vi "fpga_status.vi"(8 "error in (no error)":errorcluster, 11 "5785_2_x_200MHz in":refnum<class "5785_2_x_200MHz.lvclass">) -> (0 "error out":errorcluster, 2 "pulse TX status":T1, 3 "5785_2_x_200MHz out":refnum<class "5785_2_x_200MHz.lvclass">)   [LabVIEW 2021, in "5785_2_x_200MHz.lvclass"]
uses:
  5785_2_x_200MHz.lvclass
  5785_2_x_200MHz.lvclass/5785_2_x_200MHz.ctl
  <vilib>/Utility/error.llb/Error Cluster From Error Code.vi
  <vilib>/rvi/errors/niLvFpgaAdjustHostInterfaceError.vi
  <vilib>/rvi/interface/nirviReadWriteControl/nirviReadWriteControl.xnode
  NiFpgaLv.dll
  <vilib>/rvi/interface/Simulation/niFpgaSimulationCallBeginRW.vi
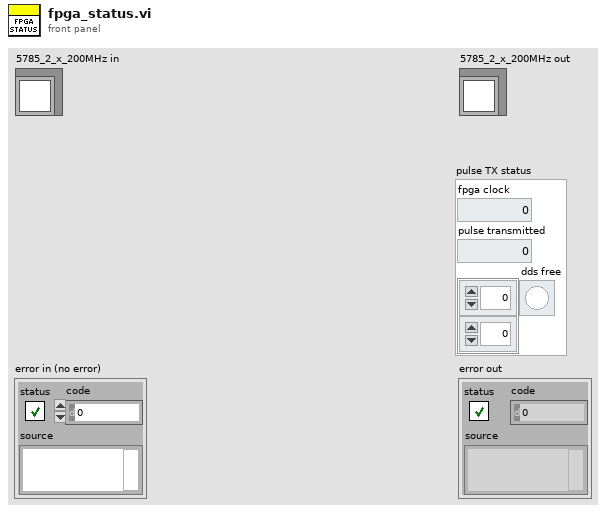
[diagram p1: front panel]
types:
  T1 = cluster{"fpga clock":dbl, "pulse transmitted":u32, "dds free":bool[][]}
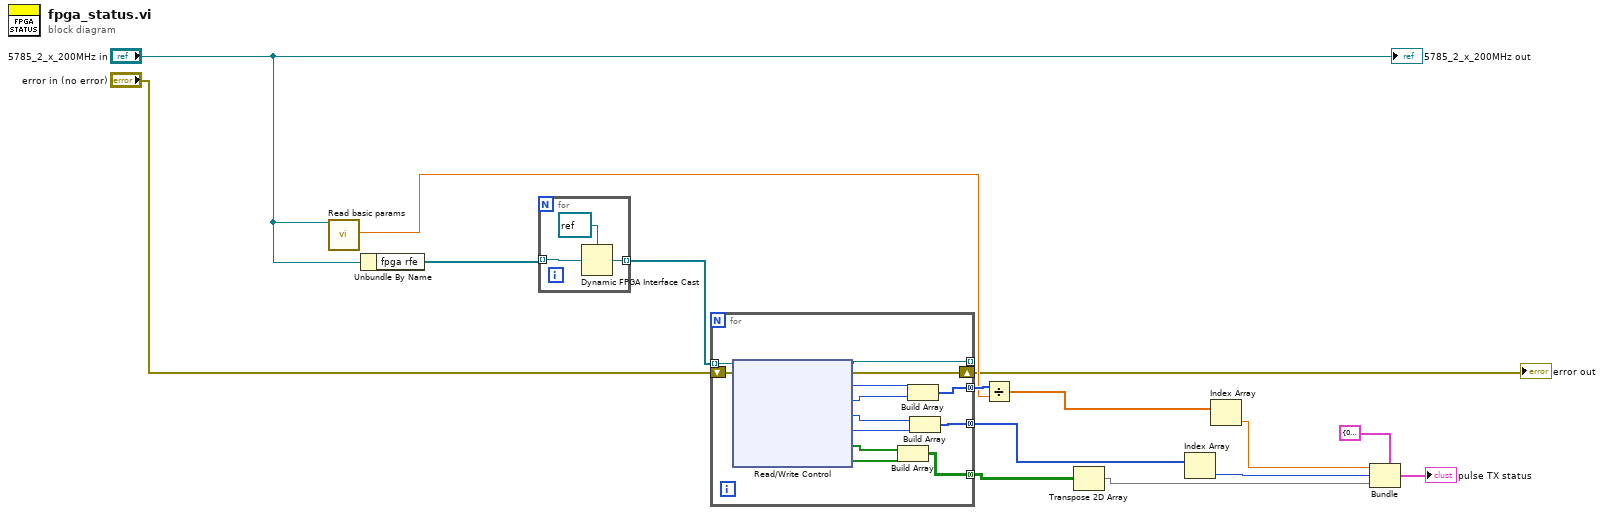
[diagram p0: block diagram]
diagram:
  n1 = call-dynamic "Read basic params.vi"("device_type in"="5785_2_x_200MHz in") -> ("Fs  FPGA"=w10:dbl)  [unwired: 13 in, 5 out]
  n2 = Unbundle By Name("5785_2_x_200MHz in") -> ("fpga rfe"=w13:refnum<k20>[])
  n3 = for {
    tunnel: w13 -> [w18] mode=indexing
    tunnel: [w16] -> w14 mode=indexing
    n4 = Dynamic FPGA Interface Cast(Session In=refnum<k20> refnum ("fpga interface out"), Type=w18) -> (Session Out=w16:refnum<k20>)
  }
  n5 = for {
    tunnel: w14 -> [w28] mode=indexing
    shift-right: [w30] -> w9
    shift-left: "error in (no error)" -> [w31]
    tunnel: [w29] -> _ mode=indexing
    tunnel: [w25] -> w12 mode=concatenating
    tunnel: [w22] -> w3 mode=concatenating
    tunnel: [w19] -> w15 mode=concatenating
    n6 = xnode "Read/Write Control"("FPGA VI Reference In"=w28, "error in"=w31) -> ("FPGA VI Reference Out"=w29:refnum<k20>, "error out"=w30:errorcluster, "fpga clock"=w21:u64, "fpga clock 2"=w20:u64, "pulse transmitted"=w24:u32, "pulse transmitted 2"=w23:u32, "dds free"=w27:bool[], "dds free 2"=w26:bool[])
    n7 = Build Array(w27, w26) -> (w25:bool[][])
    n8 = Build Array(w21, w20) -> (w19:u64[])
    n9 = Build Array(w24, w23) -> (w22:u32[])
  }
  "error out" <- w9
  n10 = Divide(x=w15, y=w10) -> (x/y=w5:dbl[])
  n11 = Transpose 2D Array(2D array=w12) -> (transposed array=w6:bool[][])
  n12 = Index Array(array=w3) -> (element=w2:u32)  [unwired: 1 in]
  n13 = Index Array(array=w5) -> (element=w4:dbl)  [unwired: 1 in]
  n14 = Bundle(cluster=T1 {"fpga clock"=0.0, "pulse transmitted"=0, "dds free"=[[FALSE, FALSE, FALSE, FALSE, FALSE, FALSE, FALSE, FALSE, FALSE, FALSE, FALSE, FALSE, FALSE, FALSE, FALSE, FALSE]]} ("pulse TX status"), "fpga clock"=w4, "pulse transmitted"=w2, "dds free"=w6) -> (→"pulse TX status":T1)
  "5785_2_x_200MHz out" <- "5785_2_x_200MHz in"
